vi "Write Command String.vi"(8 "error in (no error)":errorcluster, 10 "Command String":string, 11 "RxTxCamera in":refnum<class "RxTxCamera.lvclass">) -> (0 "error out":errorcluster, 3 "RxTxCamera out":refnum<class "RxTxCamera.lvclass">)   [LabVIEW 2018, in "RxTxCamera.lvclass"]
doc: "Este VI escreve a string do comando a ser enviado, colocando a tag CMMD na primeira linha."
uses:
  RxTxCamera.lvclass
  C:/Users/Cliente/Desktop/Software Echarpe/RxTx/RxTx.lvclass
  RxTx/RxTx.lvclass/RxTx.ctl
  RxTx/RxTx.lvclass
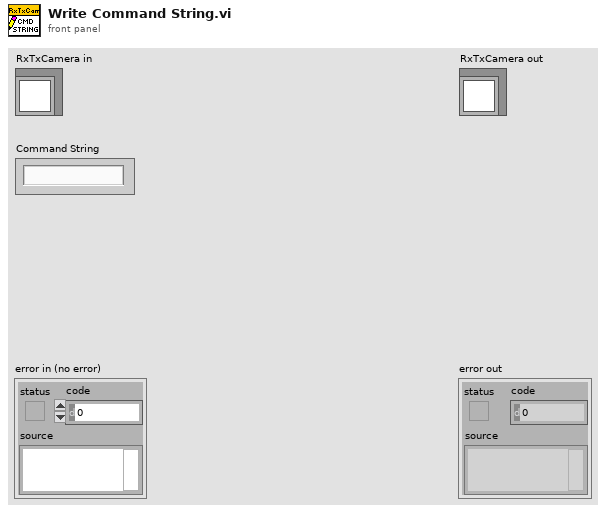
[diagram p1: front panel]
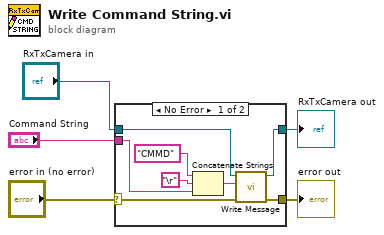
[diagram p0: block diagram]
diagram:
  n1 = case shown="No Error" "error in (no error)" {
    selector: "error in (no error)" -> [w7 w14]
    tunnel: [w6 w14] -> w4
    tunnel: [w8 w15] -> w2
    tunnel: "RxTxCamera in" -> [w9 w15]
    tunnel: "Command String" -> [w10 _]
    frame No Error {
      n2 = Concatenate Strings("CMMD", "\r", w10) -> (w11:string)
      n3 = call "Write Message.vi"("error in (no error)"=w7, "Message"=w11, "RxTx in"=w9) -> ("error out"=w6:errorcluster, "RxTx out"=w8:refnum<class "RxTxCamera.lvclass">)  [unwired: 7 in]
    }
    frame Error {
    }
  }
  "error out" <- w4
  "RxTxCamera out" <- w2
